vi "Assert.vi"(4 "Variable Y":variant, 6 "Variable X":variant, 11 "Assert Equal in":refnum<class "Assert Not Equal.lvclass">) -> (2 "Assert?":bool)   [LabVIEW 2019, in "Run Time Assertions.lvlib" / "Assert Not Equal.lvclass"]
uses:
  <vilib>/gpm_packages/@cs/run-time-assertions/Source/Assert Not Equal/Assert Not Equal.lvclass
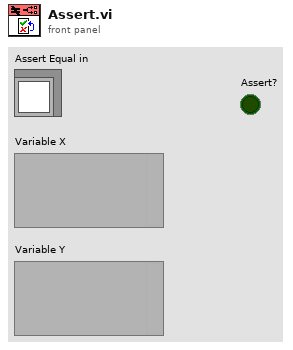
[diagram p1: front panel]
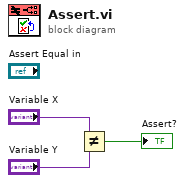
[diagram p0: block diagram]
diagram:
  n1 = Not Equal?(x="Variable X", y="Variable Y") -> (x != y?=→"Assert?":bool)
